vi "main.vi"() -> ()   [LabVIEW 2017]
panel:
  out "CH4 Pressure":dynamicdata(graph)
  in  "PID gains":T1={"proportional gain (Kc)"=1.0, "integral time (Ti, min)"=0.01, "derivative time (Td, min)"=0.0} {"derivative time (Td, min)" format="%.3f"; "integral time (Ti, min)" format="%.3f"; "proportional gain (Kc)" format="%.3f"}
  in  "CH4 Target Pressure (psi)":dbl
  out "LOX Pressure":dynamicdata(graph)
  in  "LOX Target Pressure (psi)":dbl
  in  "Regulate Pressure":bool
  in  "stop (F)":bool
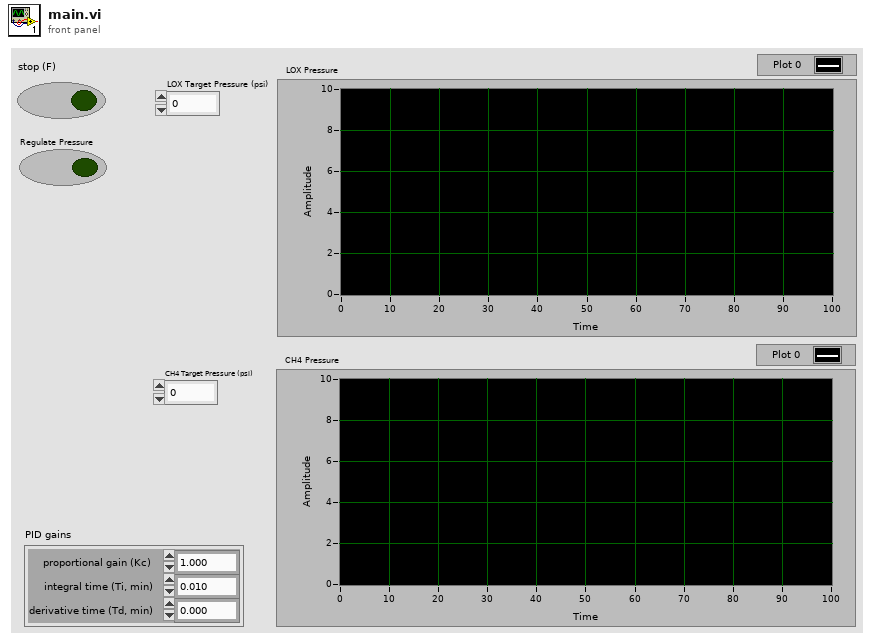
[diagram p1: front panel]
types:
  T1 = cluster{"proportional gain (Kc)":dbl, "integral time (Ti, min)":dbl, "derivative time (Td, min)":dbl}
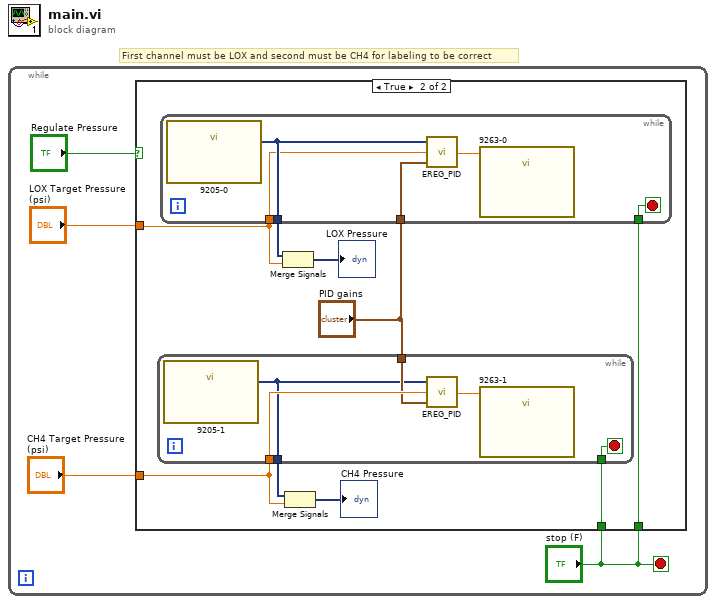
[diagram p0: block diagram]
diagram:
  # "First channel must be LOX and second must be CH4 for labeling to be correct"
  n1 = while {
    stop <- "stop (F)" stop-if-true
    n2 = case shown="True" "Regulate Pressure" {
      tunnel: "LOX Target Pressure (psi)" -> [_ w11]
      tunnel: "CH4 Target Pressure (psi)" -> [_ w8]
      tunnel: "stop (F)" -> [_ w7]
      tunnel: "stop (F)" -> [_ w6]
      frame False {
      }
      frame True {
        n3 = while {
          tunnel: [w14] -> w9
          tunnel: w8 -> [w18]
          tunnel: w7 -> [w16]
          tunnel: "PID gains" -> [w15]
          stop <- w16 stop-if-true
          n4 = call "9205-1"() -> ("data"=w14:dynamicdata)  [unwired: 17 in, 2 out]
          n5 = call "EREG_PID.vi"("PID gains"=w15, "Target Pressure (psi)"=w18, "data"=w14) -> ("Output"=w17:dbl)
          n6 = call "9263-1"("data"=w17) -> ()  [unwired: 17 in, 2 out]
        }
        n7 = while {
          tunnel: [w23] -> w12
          tunnel: w11 -> [w22]
          tunnel: w6 -> [w20]
          tunnel: "PID gains" -> [w19]
          stop <- w20 stop-if-true
          n8 = call "9205-0"() -> ("data"=w23:dynamicdata)  [unwired: 17 in, 2 out]
          n9 = call "EREG_PID.vi"("PID gains"=w19, "Target Pressure (psi)"=w22, "data"=w23) -> ("Output"=w21:dbl)
          n10 = call "9263-0"("data"=w21) -> ()  [unwired: 17 in, 2 out]
        }
        n11 = Merge Signals(w12, w11) -> (→"LOX Pressure":dynamicdata)
        n12 = Merge Signals(w9, w8) -> (→"CH4 Pressure":dynamicdata)
      }
    }
  }
